vi "ServiceModeTest1.vi"(0 "GEA2 Reference In":refnum<k24>, 1 "Faults ON ERD Array":T1[](array[typedef])=[{"ERD Number"=64912, "Data Type"=enum."string", "Data"="01"}, {"ERD Number"=64913, "Data Type"=enum."string", "Data"="01"}, {"ERD Number"=64914, "Data Type"=enum."string", "Data"="01"}, {"ERD Number"=64915, "Data Type"=enum."string", "Data"="01"}, {"ERD Number"=64916, "Data Type"=enum."string", "Data"="01"}, {"ERD Number"=64917, "Data Type"=enum."string", "Data"="01"}, {"ERD Number"=64918, "Data Type"=enum."string", "Data"="01"}, {"ERD Number"=64919, "Data Type"=enum."string", "Data"="01"}, {"ERD Number"=64920, "Data Type"=enum."string", "Data"="01"}, {"ERD Number"=64921, "Data Type"=enum."string", "Data"="01"}] {"ERD Number" format="%.0x"}, 5 "MC GEA Inputs":T3={"Source"=228, "Destination"=36} {"Destination" format="%.0x"; "Source" format="%.0x"}, 7 "UI GEA Inputs":T3={"Source"=228, "Destination"=37} {"Destination" format="%.0x"; "Source" format="%.0x"}, 9 "Erd_ServiceDiagnosticsFaultTableClear ERD #":T1={"ERD Number"=57604, "Data Type"=enum."string", "Data"="01"} {"ERD Number" format="%.0x"}, 11 "Error In":errorcluster, 12 "Faults OFF ERD Array":T1[](array[typedef])=[{"ERD Number"=64912, "Data Type"=enum."string", "Data"="00"}, {"ERD Number"=64913, "Data Type"=enum."string", "Data"="00"}, {"ERD Number"=64914, "Data Type"=enum."string", "Data"="00"}, {"ERD Number"=64915, "Data Type"=enum."string", "Data"="00"}, {"ERD Number"=64916, "Data Type"=enum."string", "Data"="00"}, {"ERD Number"=64917, "Data Type"=enum."string", "Data"="00"}, {"ERD Number"=64918, "Data Type"=enum."string", "Data"="00"}, {"ERD Number"=64919, "Data Type"=enum."string", "Data"="00"}, {"ERD Number"=64920, "Data Type"=enum."string", "Data"="00"}, {"ERD Number"=64921, "Data Type"=enum."string", "Data"="00"}] {"ERD Number" format="%.0x"}) -> (4 "GEA2 Reference Out":refnum<k24>, 6 "Pass/Fail?":bool, 8 "Report Text":string, 15 "Error Out":errorcluster)   [LabVIEW 2016]
uses:
  Q:/Common/DLLs/GEA3/GeaCommunication.dll
  Common/DLLs/GEA3/GeaCommunication.dll
  Common/LabVIEW GEA2 Toolkit/LabVIEW_GEA2_Toolkit.lvlibp/type defs/Source_Destination.ctl
  Common/LabVIEW GEA2 Toolkit/LabVIEW_GEA2_Toolkit.lvlibp/type defs/ERD Write Data In.ctl
  Common/LabVIEW GEA2 Toolkit/LabVIEW_GEA2_Toolkit.lvlibp/type defs/Data Type.ctl
  Centauro Washer/Product Testcode/Centauro/Valew Common/type defs/LED Status OOB.ctl
  Common/Type Defs/JL_Buttons.ctl
  Common/LabVIEW GEA2 Toolkit/LabVIEW_GEA2_Toolkit.lvlibp
panel:
  in  "Board Index":i32
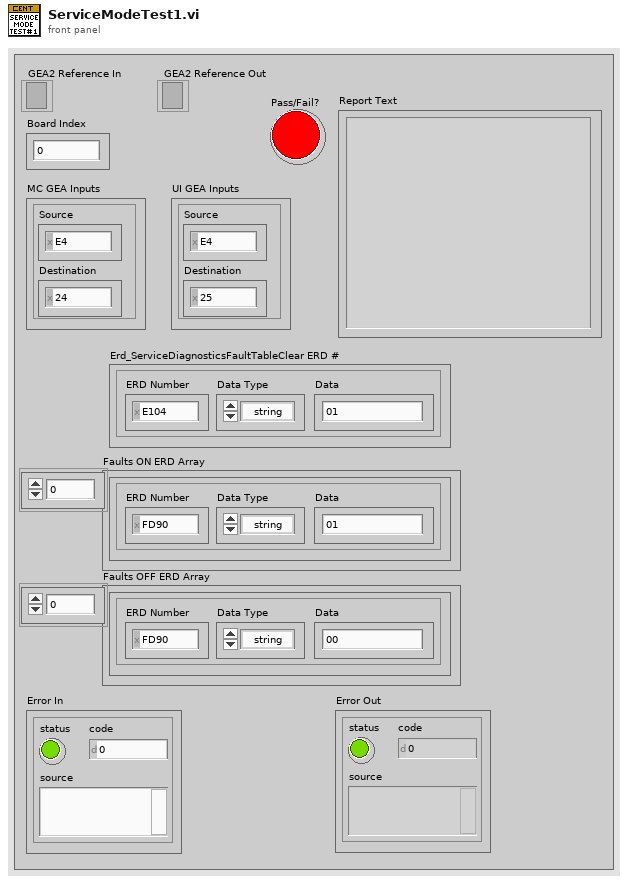
[diagram p1: front panel]
types:
  T1 = typedef "LabVIEW_GEA2_Toolkit.lvlibp/ERD Write Data In.ctl" = cluster{"ERD Number":u16, "Data Type":T2, "Data":string}
  T2 = typedef "LabVIEW_GEA2_Toolkit.lvlibp/Data Type.ctl" = enum16{"string", "boolean", "uint8_t", "uint16_t", "uint32_t", "uint64_t", "int8_t", "int16_t", "int32_t", "int64_t"}
  T3 = typedef "LabVIEW_GEA2_Toolkit.lvlibp/Source_Destination.ctl" = cluster{"Source":u8, "Destination":u8}
  T4 = typedef "JL_Buttons.ctl" = enum16{"Power", "Start / Pause ", "Temp Option ", "Dryness Level", "Time Option", "Time Increment ", "Time Decrement ", "MyCycle", "eDry ", "Delay", "Extended Tumble", "Control Lock", "Volume/Signal", "Damp Alert / Drum Light", "Unused", "(SW213)", "(SW322)", "Clear / Reset"}
  T5 = typedef "LED Status OOB.ctl" = enum32{"Off", "On", "Blink"}
  T6 = cluster{"Damp":T5, "Dry":T5, "Cool":T5, "Eco":T5}
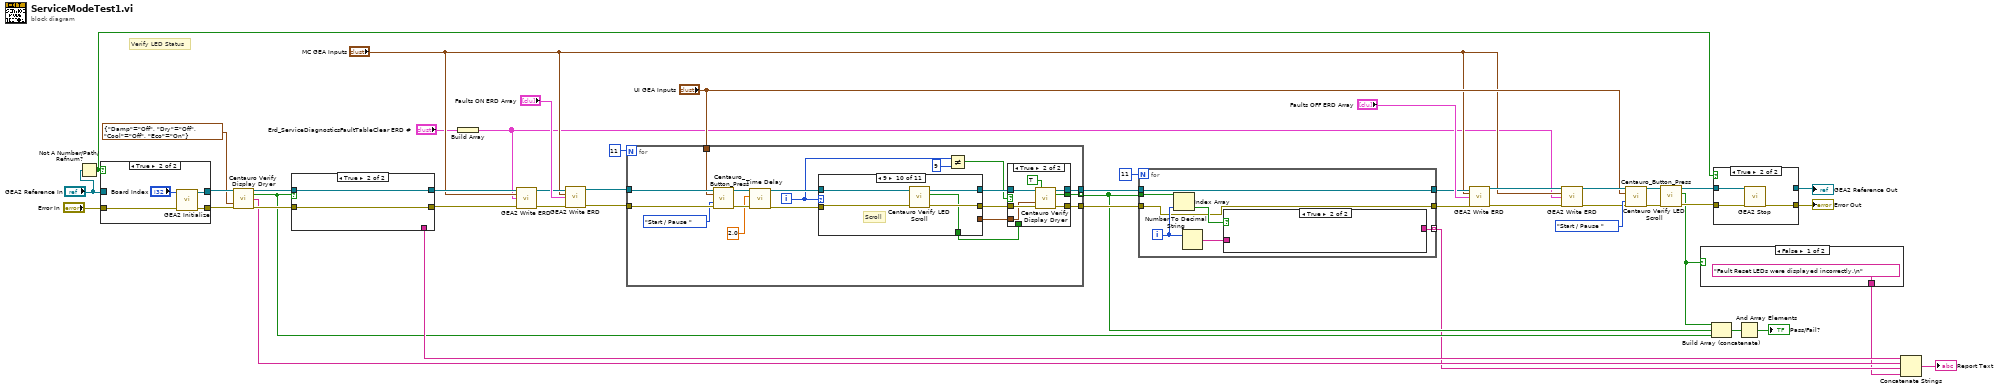
[diagram p0: block diagram]
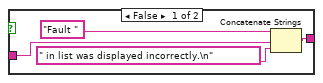
[diagram p4: hidden frame]
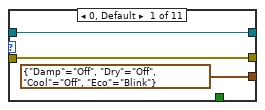
[diagram p6: hidden frame]
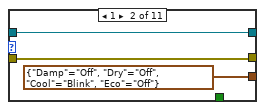
[diagram p7: hidden frame]
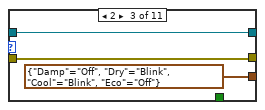
[diagram p8: hidden frame]
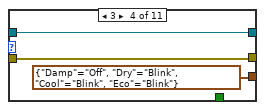
[diagram p9: hidden frame]
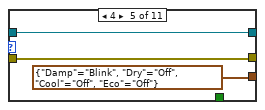
[diagram p10: hidden frame]
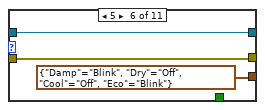
[diagram p11: hidden frame]
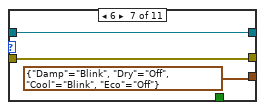
[diagram p12: hidden frame]
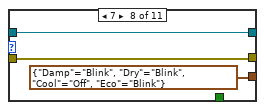
[diagram p13: hidden frame]
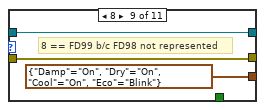
[diagram p14: hidden frame]
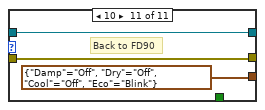
[diagram p15: hidden frame]
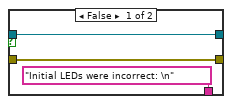
[diagram p16: hidden frame]
diagram:
  # "Verify LED Status"
  n1 = Not A Number/Path/Refnum?(number/path/refnum="GEA2 Reference In") -> (NaN/Path/Refnum?=w5:bool)
  n2 = case shown="True" w5 {
    tunnel: [w48 w53] -> w45
    tunnel: "Error In" -> [w48 w52]
    tunnel: [w49 w51] -> w46
    tunnel: "GEA2 Reference In" -> [w49 _]
    frame False {
    }
    frame True {
      n3 = call "GEA2 Initialize.vi"("Board Index"="Board Index", "error in"=w52) -> ("GEA2 Reference Out"=w51:refnum<k24>, "error out"=w53:errorcluster)  [unwired: 11 in, 1 out]
    }
  }
  n4 = call "Centauro Verify Display Dryer.vi"("GEA2 Reference In"=w46, "Expected LED Status"=T6 {"Damp"=enum."Off", "Dry"=enum."Off", "Cool"=enum."Off", "Eco"=enum."On"}, "Error In"=w45) -> ("GEA2 Reference Out"=w44:refnum<k24>, "Pass/Fail?"=w25:bool, "Report Text"=w40:string, "Error Out"=w43:errorcluster)  [unwired: 7 in, 2 out]
  n5 = case shown="True" w25 {
    tunnel: w44 -> [w56 w58]
    tunnel: [w56 w58] -> w15
    tunnel: [w55 w57] -> w13
    tunnel: w43 -> [w55 w57]
    tunnel: ["Initial LEDs were incorrect: \n" _] -> w41
    frame False {
    }
    frame True {
    }
  }
  n6 = Build Array("Erd_ServiceDiagnosticsFaultTableClear ERD #") -> (w1:T1[])
  n7 = call "GEA2 Write ERD.vi"("GEA2 Reference In"=w15, "GEA Inputs"="MC GEA Inputs", "Write ERD List"=w1, "Error In"=w13) -> ("GEA2 Reference Out"=w14:refnum<k24>, "Error Out"=w12:errorcluster)  [unwired: 9 in, 1 out]
  n8 = call "GEA2 Write ERD.vi"("GEA2 Reference In"=w14, "GEA Inputs"="MC GEA Inputs", "Write ERD List"="Faults ON ERD Array", "Error In"=w12) -> ("GEA2 Reference Out"=w37:refnum<k24>, "Error Out"=w36:errorcluster)  [unwired: 9 in, 1 out]
  n9 = for {
    N: 11 -> [_]
    tunnel: w37 -> [w76]
    tunnel: w36 -> [w75]
    tunnel: [w69] -> w26 mode=indexing
    tunnel: [w65] -> w33
    tunnel: [w64] -> w30
    tunnel: "UI GEA Inputs" -> [w63]
    i -> [w62]
    n10 = call "Centauro_Button_Press.vi"("GEA2 Reference In"=w76, "GEA Inputs"=w63, "Button"=JL_Buttons."Start / Pause ", "Error In"=w75) -> ("GEA2 Reference Out"=w72:refnum<k24>, "Error Out"=w61:errorcluster)  [unwired: 10 in]
    n11 = call "Time Delay"("error in (no error)"=w61, "Delay Time (s)"=2.0) -> ("error out"=w60:errorcluster)  [unwired: 9 in]
    n12 = case shown="9" w62 {
      tunnel: [w89 w92 w95 w98 w101 w104 w107 w110 w113 w117 w121] -> w73
      tunnel: w72 -> [w89 w92 w95 w98 w101 w104 w107 w110 w113 w118 w121]
      tunnel: [w88 w91 w94 w97 w100 w103 w106 w109 w112 w116 w120] -> w71
      tunnel: w60 -> [w88 w91 w94 w97 w100 w103 w106 w109 w112 w115 w120]
      tunnel: [T6 {"Damp"=enum."Off", "Dry"=enum."Off", "Cool"=enum."Off", "Eco"=enum."Blink"} ("Expected LED Status") T6 {"Damp"=enum."Off", "Dry"=enum."Off", "Cool"=enum."Blink", "Eco"=enum."Off"} ("Expected LED Status") T6 {"Damp"=enum."Off", "Dry"=enum."Blink", "Cool"=enum."Blink", "Eco"=enum."Off"} ("Expected LED Status") T6 {"Damp"=enum."Off", "Dry"=enum."Blink", "Cool"=enum."Blink", "Eco"=enum."Blink"} ("Expected LED Status") T6 {"Damp"=enum."Blink", "Dry"=enum."Off", "Cool"=enum."Off", "Eco"=enum."Off"} ("Expected LED Status") T6 {"Damp"=enum."Blink", "Dry"=enum."Off", "Cool"=enum."Off", "Eco"=enum."Blink"} ("Expected LED Status") T6 {"Damp"=enum."Blink", "Dry"=enum."Off", "Cool"=enum."Blink", "Eco"=enum."Off"} ("Expected LED Status") T6 {"Damp"=enum."Blink", "Dry"=enum."Blink", "Cool"=enum."Off", "Eco"=enum."Blink"} ("Expected LED Status") T6 {"Damp"=enum."On", "Dry"=enum."On", "Cool"=enum."On", "Eco"=enum."Blink"} ("Expected LED Status") _ T6 {"Damp"=enum."Off", "Dry"=enum."Off", "Cool"=enum."Off", "Eco"=enum."Blink"} ("Expected LED Status")] -> w70
      tunnel: [_ _ _ _ _ _ _ _ _ w114 _] -> w66
      frame 0, Default {
      }
      frame 1 {
      }
      frame 2 {
      }
      frame 3 {
      }
      frame 4 {
      }
      frame 5 {
      }
      frame 6 {
      }
      frame 7 {
      }
      frame 8 {
        # "8 == FD99 b/c FD98 not represented"
      }
      frame 9 {
        # "Scroll"
        n13 = call "Centauro Verify LED Scroll.vi"("Error In"=w115, "GEA2 Reference In"=w118) -> ("Error Out"=w116:errorcluster, "Pass/Fail?"=w114:bool, "GEA2 Reference Out"=w117:refnum<k24>)  [unwired: 7 in]
      }
      frame 10 {
        # "Back to FD90"
      }
    }
    n14 = Not Equal?(x=w62, y=9) -> (x != y?=w67:bool)
    n15 = case shown="True" w67 {
      tunnel: w73 -> [w78 w86]
      tunnel: w71 -> [w77 w85]
      tunnel: w70 -> [_ w81]
      tunnel: [w79 w84] -> w69
      tunnel: w66 -> [w79 _]
      tunnel: [w78 w83] -> w65
      tunnel: [w77 w82] -> w64
      frame False {
      }
      frame True {
        n16 = call "Centauro Verify Display Dryer.vi"("GEA2 Reference In"=w86, "Service Mode?"=TRUE, "Expected LED Status"=w81, "Error In"=w85) -> ("GEA2 Reference Out"=w83:refnum<k24>, "Pass/Fail?"=w84:bool, "Error Out"=w82:errorcluster)  [unwired: 6 in, 3 out]
      }
    }
  }
  n17 = for {
    N: 11 -> [_]
    tunnel: w26 -> [w128]
    tunnel: [w124] -> w18 mode=indexing
    tunnel: w33 -> [w123]
    tunnel: [w123] -> w32
    tunnel: [w122] -> w31
    tunnel: w30 -> [w122]
    i -> [w126]
    n18 = Index Array(array=w128, index=w126) -> (element=w127:bool)
    n19 = Number To Decimal String(number=w126) -> (decimal integer string=w125:string)  [unwired: 1 in]
    n20 = case shown="True" w127 {
      tunnel: w125 -> [w131 _]
      tunnel: [w129 _] -> w124
      frame False {
        n21 = Concatenate Strings("Fault ", w131, " in list was displayed incorrectly.\n") -> (w129:string)
      }
      frame True {
      }
    }
  }
  n22 = call "GEA2 Write ERD.vi"("GEA2 Reference In"=w32, "GEA Inputs"="MC GEA Inputs", "Write ERD List"="Faults OFF ERD Array", "Error In"=w31) -> ("GEA2 Reference Out"=w7:refnum<k24>, "Error Out"=w11:errorcluster)  [unwired: 9 in, 1 out]
  n23 = call "GEA2 Write ERD.vi"("GEA2 Reference In"=w7, "GEA Inputs"="MC GEA Inputs", "Write ERD List"=w1, "Error In"=w11) -> ("GEA2 Reference Out"=w10:refnum<k24>, "Error Out"=w9:errorcluster)  [unwired: 9 in, 1 out]
  n24 = call "Centauro_Button_Press.vi"("GEA2 Reference In"=w10, "GEA Inputs"="UI GEA Inputs", "Button"=JL_Buttons."Start / Pause ", "Error In"=w9) -> ("GEA2 Reference Out"=w27:refnum<k24>, "Error Out"=w28:errorcluster)  [unwired: 10 in]
  n25 = call "Centauro Verify LED Scroll.vi"("Error In"=w28, "GEA2 Reference In"=w27) -> ("Error Out"=w20:errorcluster, "Pass/Fail?"=w17:bool, "GEA2 Reference Out"=w19:refnum<k24>)  [unwired: 7 in]
  n26 = case shown="False" w17 {
    tunnel: ["Fault Reset LEDs were displayed incorrectly.\n" _] -> w16
    frame False {
    }
    frame True {
    }
  }
  n27 = Build Array (concatenate)(w17, w26, w25) -> (w24:bool[])
  n28 = case shown="True" w5 {
    tunnel: [w134 w138] -> w22
    tunnel: w19 -> [w135 w137]
    tunnel: w20 -> [w134 w136]
    tunnel: [w135 _] -> w21
    frame False {
    }
    frame True {
      n29 = call "GEA2 Stop.vi"("GEA2 Reference In"=w137, "Error In"=w136) -> ("Error Out"=w138:errorcluster)  [unwired: 13 in]
    }
  }
  "GEA2 Reference Out" <- w21
  "Error Out" <- w22
  n30 = And Array Elements(Boolean array=w24) -> (logical AND=→"Pass/Fail?":bool)
  n31 = Concatenate Strings(w41, w40, w18, w16) -> (→"Report Text":string)
